vi "Queue read.vi"(8 "Error in (no error)":errorcluster caption="error out（no error）", 11 "Queue Input":refnum<queue>) -> (0 "Error out":errorcluster caption="error out", 1 "Timeout？":bool, 2 "Output Array":sgl[](array[numeric]))   [LabVIEW 2019]
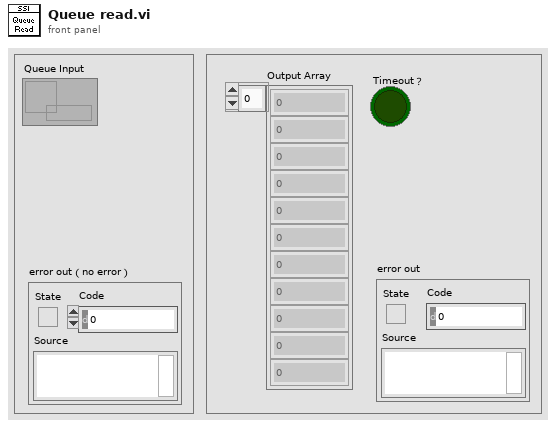
[diagram p1: front panel]
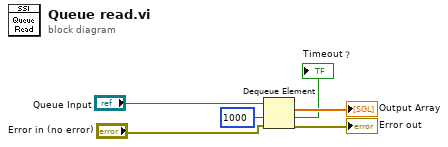
[diagram p0: block diagram]
diagram:
  n1 = Dequeue Element(queue="Queue Input", timeout in ms (-1)=1000 ("超时毫秒(-1)"), error in (no error)="Error in (no error)") -> (element=→"Output Array":sgl[], timed out?=→"Timeout？":bool, error out=→"Error out":errorcluster)  [unwired: 1 out]
